vi "toString.vi"(8 "error in (no error)":errorcluster, 11 "Composite Employee in":refnum<class "Composite Employee.lvclass">) -> (0 "error out":errorcluster, 2 "resulting string":string, 3 "Composite Employee out":refnum<class "Composite Employee.lvclass">)   [LabVIEW 2017, in "Composite Employee.lvclass"]
uses:
  Composite Employee.lvclass
  Composite Employee.lvclass/Composite Employee.ctl
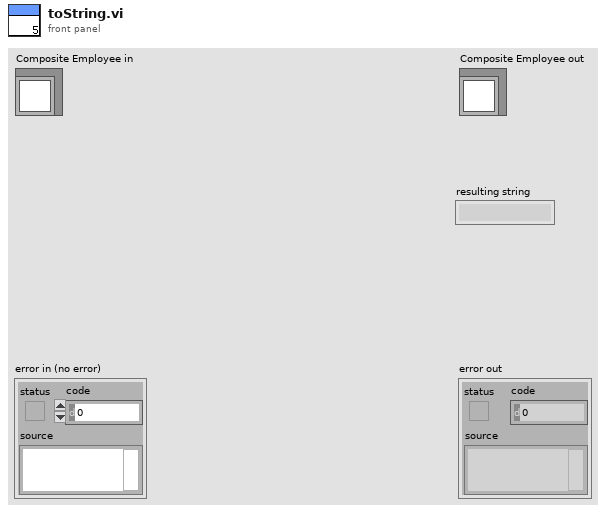
[diagram p1: front panel]
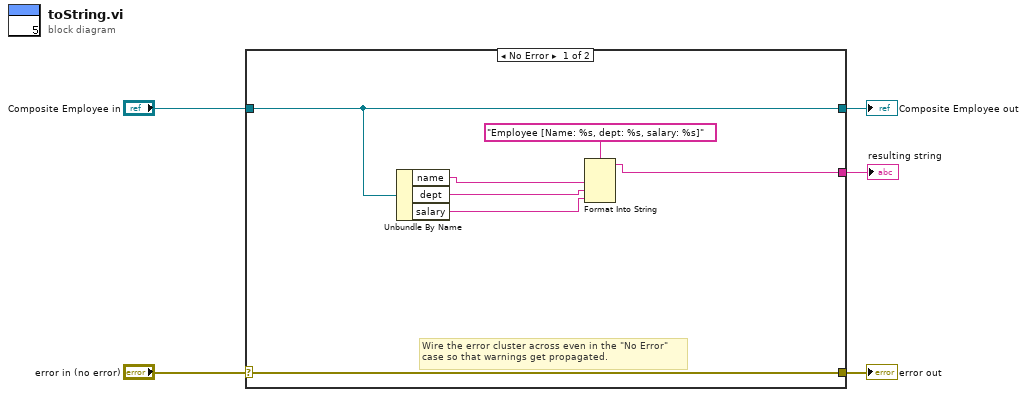
[diagram p0: block diagram]
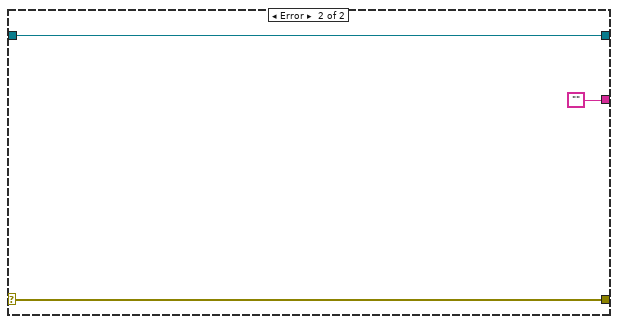
[diagram p2: hidden frame]
diagram:
  n1 = case shown="No Error" "error in (no error)" {
    selector: "error in (no error)" -> [w12 w15]
    tunnel: [w12 w15] -> w4
    tunnel: [w11 w14] -> w2
    tunnel: "Composite Employee in" -> [w11 w14]
    tunnel: [w6 ""] -> w1
    frame No Error {
      # "Wire the error cluster across even in the \"No Error\"\ncase so that warnings get propagated."
      n2 = Unbundle By Name(w11) -> ("name"=w9:string, "dept"=w8:string, "salary"=w7:string)
      n3 = Format Into String(format string="Employee [Name: %s, dept: %s, salary: %s]", w9, w8, w7) -> (resulting string=w6:string)  [unwired: 2 in, 1 out]
    }
    frame Error {
    }
  }
  "error out" <- w4
  "Composite Employee out" <- w2
  "resulting string" <- w1
